vi "hla_obj_to_log_entry.vi"(10 "obj":T1) -> (2 "entry (out)":string)   [LabVIEW 2016]
uses:
  controls/hla_queue_obj.ctl
  controls/hla_param.ctl
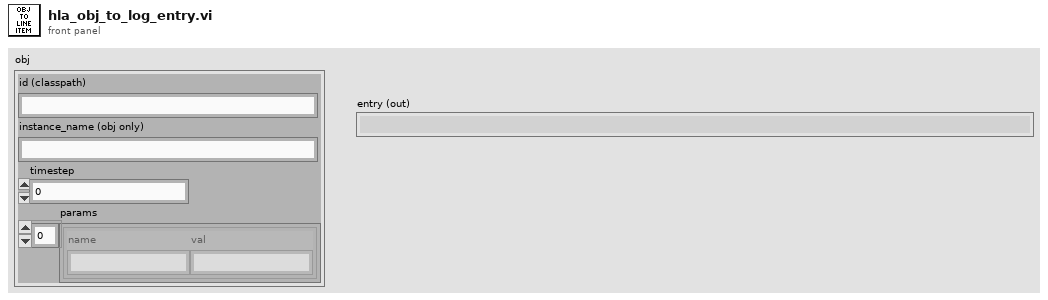
[diagram p1: front panel]
types:
  T1 = typedef "hla_queue_obj.ctl" = cluster{"id (classpath)":string, "instance_name (obj only)":string, "timestep":dbl, "params":T2[]}
  T2 = typedef "hla_param.ctl" = cluster{"name":string, "val":string}
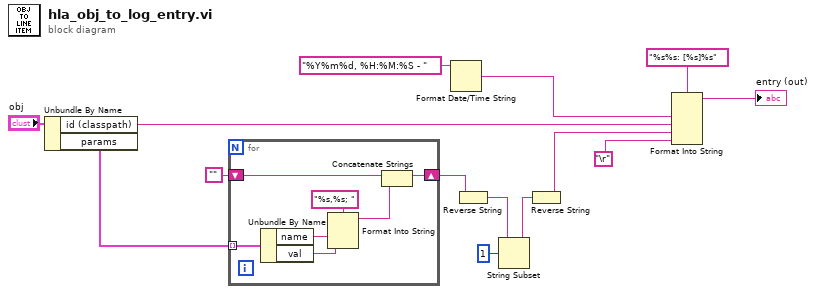
[diagram p0: block diagram]
diagram:
  n1 = Unbundle By Name("obj") -> ("id (classpath)"=w2:string, "params"=w13:T2[])
  n2 = for {
    tunnel: w13 -> [w21] mode=indexing
    shift-right: [w15] -> w5
    shift-left: "" -> [w17]
    n3 = Unbundle By Name(w21) -> ("name"=w19:string, "val"=w18:string)
    n4 = Format Into String(format string="%s,%s; ", w19, w18) -> (resulting string=w16:string)  [unwired: 2 in, 1 out]
    n5 = Concatenate Strings(w17, w16) -> (w15:string)
  }
  n6 = Format Date/Time String(time format string (%c)="%Y%m%d, %H:%M:%S - ") -> (date/time string=w1:string)  [unwired: 2 in]
  n7 = Reverse String(1:w5) -> (0:w8:string)
  n8 = String Subset(string=w8, offset (0)=1) -> (substring=w6:string)  [unwired: 1 in]
  n9 = Reverse String(1:w6) -> (0:w4:string)
  n10 = Format Into String(format string="%s%s: [%s]%s", w1, w2, w4, "\r") -> (resulting string=→"entry (out)":string)  [unwired: 2 in, 1 out]
